vi "QuickCheckStop.vi"(8 "error in (no error)":errorcluster, 11 "Tapedrive Object":refnum<class "Tapedrive_ESP301.lvclass">) -> (0 "error out (no error)":errorcluster, 2 "new commands":string, 3 "Tapedrive Object 2":refnum<class "Tapedrive_ESP301.lvclass">)   [LabVIEW 2013, in "Tapedrive_ESP301.lvclass"]
uses:
  Tapedrive_ESP301.lvclass
panel:
  out "Position (units)":dbl(graph)
  out "Velocity (units/s)":dbl(graph)
  out "Waveform Graph 2":dbl[][](graph)
  out "Waveform Graph":dbl[](graph)
  out "Numeric":i32
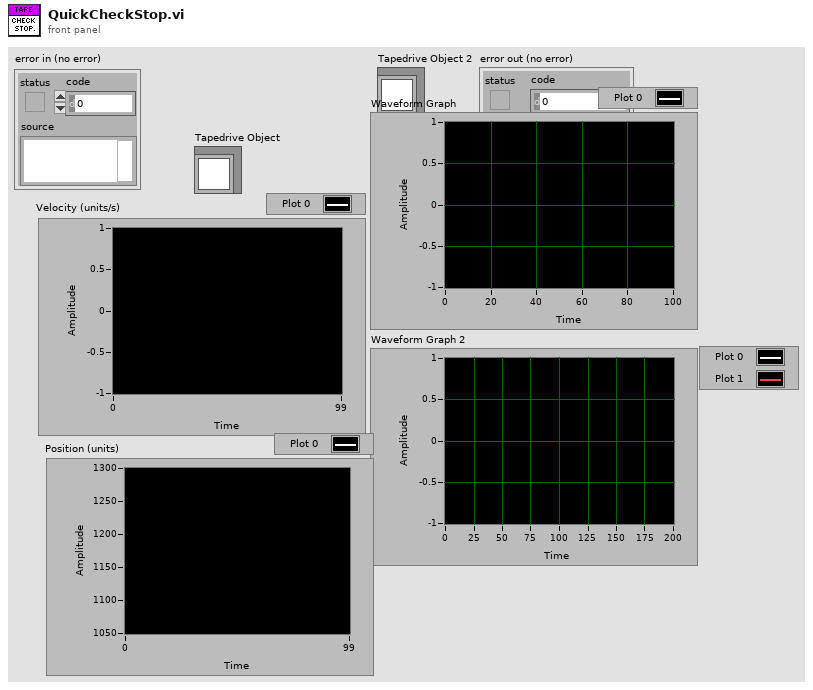
[diagram p1: front panel]
types:
  T1 = typedef "Direction.ctl" = enum16{"Forward", "Backward", "Undefined"}
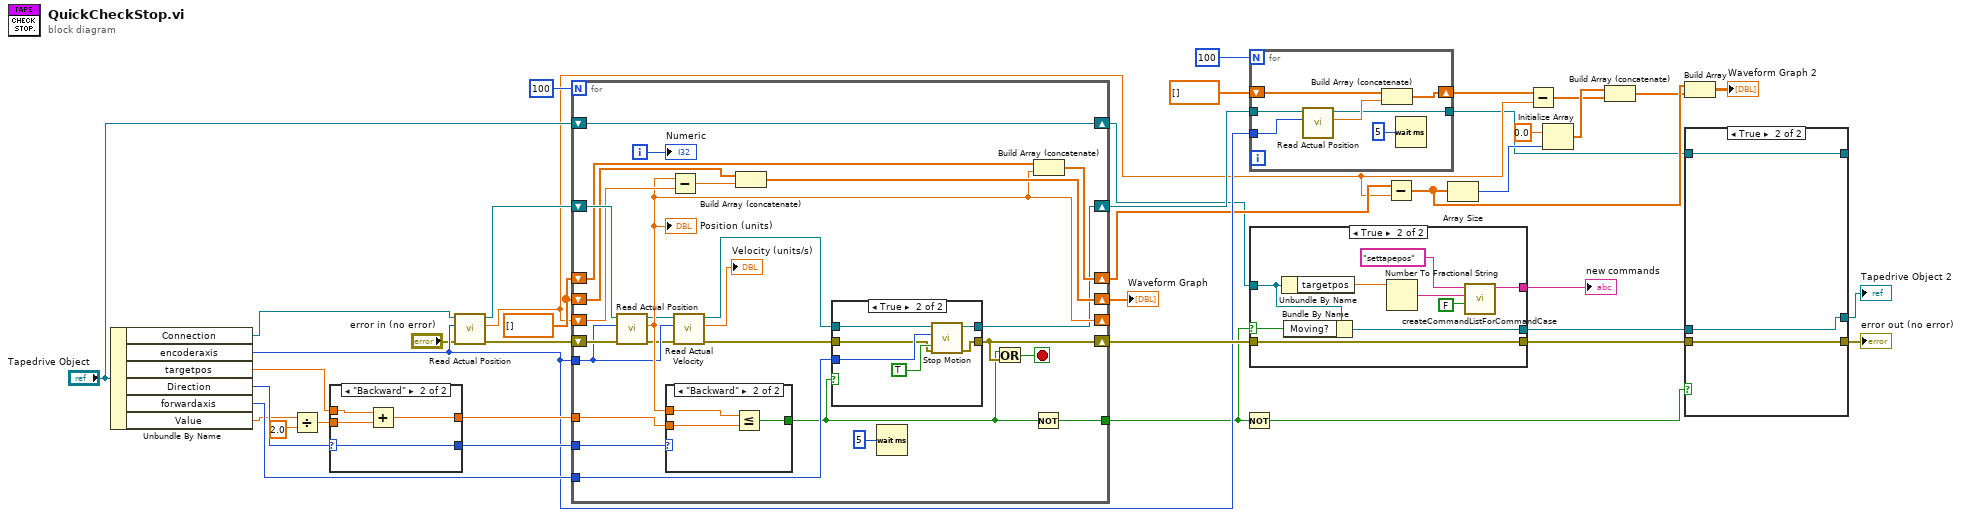
[diagram p0: block diagram]
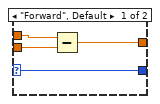
[diagram p3: hidden frame]
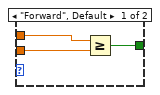
[diagram p6: hidden frame]
diagram:
  w29 = dbl[] []
  n1 = Unbundle By Name("Tapedrive Object") -> ("Connection"=w32:refnum<visa-resource-name>, "encoderaxis"=w26:i16, "targetpos"=w36:dbl, "Direction"=w37:T1, "forwardaxis"=w33:i16, "Value"=w24:dbl)
  n2 = Divide(x=w24, y=2.0) -> (x/y=w22:dbl)
  n3 = case shown="\"Backward\"" w37 {
    selector: w37 -> [w44 w48]
    tunnel: w36 -> [w43 w47]
    tunnel: [w44 w48] -> w35
    tunnel: w22 -> [w42 w46]
    tunnel: [w41 w45] -> w34
    frame "Forward", Default {
      n4 = Subtract(x=w43, y=w42) -> (x-y=w41:dbl)
    }
    frame "Backward" {
      n5 = Add(x=w47, y=w46) -> (x+y=w45:dbl)
    }
  }
  n6 = call <instrlib>:"Read Actual Position.vi"("error in (no error)"="error in (no error)", "Axis (1)"=w26, "VISA resource name"=w32) -> ("error out"=w1:errorcluster, "Position (units)"=w20:dbl, "VISA resource name out"=w31:refnum<visa-resource-name>)  [unwired: 2 in]
  n7 = for {
    N: 100 -> [_]
    shift-right: [w71] -> w10
    shift-left: "Tapedrive Object" -> [w71]
    tunnel: w26 -> [w52]
    shift-right: [w64] -> w38
    shift-left: w1 -> [w72]
    tunnel: [w68] -> w6
    tunnel: w35 -> [w67]
    tunnel: w34 -> [w66]
    tunnel: w33 -> [w65]
    shift-right: [w57] -> _
    shift-left: w20 -> [w62]
    shift-right: [w60] -> w30
    shift-left: w29 -> [w59]
    shift-right: [w56] -> w21
    shift-left: w29 -> [w58]
    shift-right: [w55] -> w27
    shift-left: w31 -> [w73]
    i -> [w69]
    stop <- w74 stop-if-true
    n8 = call <instrlib>:"Read Actual Position.vi"("error in (no error)"=w72, "Axis (1)"=w52, "VISA resource name"=w73) -> ("error out"=w50:errorcluster, "Position (units)"=w57:dbl, "VISA resource name out"=w54:refnum<visa-resource-name>)  [unwired: 2 in]
    "Position (units)" <- w57
    n9 = case shown="\"Backward\"" w67 {
      tunnel: w66 -> [w84 w87]
      tunnel: w57 -> [w85 w88]
      tunnel: [w83 w86] -> w63
      frame "Forward", Default {
        n10 = Greater Or Equal?(x=w85, y=w84) -> (x >= y?=w83:bool)
      }
      frame "Backward" {
        n11 = Less Or Equal?(x=w88, y=w87) -> (x <= y?=w86:bool)
      }
    }
    n12 = Subtract(x=w57, y=w62) -> (x-y=w61:dbl)
    n13 = call <instrlib>:"Read Actual Velocity.vi"("error in (no error)"=w50, "Axis (1)"=w52, "VISA resource name"=w54) -> ("error out"=w49:errorcluster, "Velocity (units/s)"=→"Velocity (units/s)":dbl, "VISA resource name out"=w53:refnum<visa-resource-name>)  [unwired: 2 in]
    n14 = Build Array (concatenate)(w59, w61) -> (w60:dbl[])
    n15 = case shown="True" w63 {
      tunnel: w53 -> [w75 w82]
      tunnel: w65 -> [_ w81]
      tunnel: w49 -> [w76 w79]
      tunnel: [w76 w78] -> w64
      tunnel: [w75 w77] -> w55
      frame False {
      }
      frame True {
        n16 = call <instrlib>:"Stop Motion.vi"("error in (no error)"=w79, "Stop all axes (F)"=TRUE, "Axis (1)"=w81, "VISA resource name"=w82) -> ("error out"=w78:errorcluster, "VISA resource name out"=w77:refnum<visa-resource-name>)  [unwired: 2 in]
      }
    }
    n17 = Wait (ms)(milliseconds to wait=u32 5) -> ()  [unwired: 1 out]
    n18 = Or(x=w63, y=w64) -> (x .or. y?=w74:bool)
    n19 = Not(x=w63) -> (.not. x?=w68:bool)
    n20 = Build Array (concatenate)(w58, w57) -> (w56:dbl[])
    "Numeric" <- w69
  }
  "Waveform Graph" <- w30
  n21 = Not(x=w6) -> (.not. x?=w5:bool)
  n22 = for {
    N: 100 -> [_]
    tunnel: w27 -> [w94]
    tunnel: w26 -> [w93]
    shift-right: [w91] -> w25
    shift-left: dbl[] [] -> [w90]
    tunnel: [w89] -> w11
    n23 = call <instrlib>:"Read Actual Position.vi"("Axis (1)"=w93, "VISA resource name"=w94) -> ("Position (units)"=w92:dbl, "VISA resource name out"=w89:refnum<visa-resource-name>)  [unwired: 3 in, 1 out]
    n24 = Build Array (concatenate)(w90, w92) -> (w91:dbl[])
    n25 = Wait (ms)(milliseconds to wait=u32 5) -> ()  [unwired: 1 out]
  }
  n26 = case shown="True" w6 {
    selector: w6 -> [_ w100]
    tunnel: w38 -> [w97 w106]
    tunnel: [w97 w106] -> w7
    tunnel: [w96 w99] -> w12
    tunnel: w10 -> [w96 w101]
    tunnel: [_ w98] -> w3
    frame False {
    }
    frame True {
      n27 = Unbundle By Name(w101) -> ("targetpos"=w103:dbl)
      n28 = Bundle By Name(cluster=w101, "Moving?"=w100) -> (w99:refnum<class "Tapedrive_ESP301.lvclass">)
      n29 = Number To Fractional String(number=w103) -> (F-format string=w102:string)  [unwired: 3 in]
      n30 = call "createCommandListForCommandCase.vi"("immediate Check (only once)"=FALSE, "setvalue"=w102, "command"="settapepos") -> ("new commands"=w98:string)  [unwired: 8 in]
    }
  }
  "new commands" <- w3
  n31 = Subtract(x=w21, y=w20) -> (x-y=w18:dbl[])
  n32 = Array Size(array=w18) -> (size(s)=w17:i32)
  n33 = Subtract(x=w25, y=w20) -> (x-y=w14:dbl[])
  n34 = Initialize Array(0.0 ("element"), w17) -> (w15:dbl[])
  n35 = Build Array (concatenate)(w15, w14) -> (w13:dbl[])
  n36 = Build Array(w18, w13) -> (→"Waveform Graph 2":dbl[][])
  n37 = case shown="True" w5 {
    tunnel: w12 -> [w108 w112]
    tunnel: w7 -> [w107 w111]
    tunnel: [w107 w111] -> w4
    tunnel: [w108 w112] -> w9
    tunnel: w11 -> [w109 w110]
    tunnel: [w109 w110] -> _
    frame False {
    }
    frame True {
    }
  }
  "Tapedrive Object 2" <- w9
  "error out (no error)" <- w4
